vi "Async Engine.vi"(10 "Parameters":variant, 11 "Process":refnum<class "Process.lvclass">) -> ()   [LabVIEW 2019, in "Fuel Injector Analysis Addon Engine.lvlib"]
uses:
  Fuel Injector Analysis Addon Engine.lvlib
  <vilib>/NI/NIVS Inline Async API/_VS Inline Async API/Process/Process.lvclass
  Addon Shared/Types/Injector info.ctl
  Addon Shared/Fuel Injector Analysis Addon Shared.lvlib
  <vilib>/NI VeriStand/Custom Device API/Waveform Data Reference.ctl
  <vilib>/NI VeriStand/Custom Device API/Custom Device API.lvlib
  <vilib>/NI VeriStand/Custom Device Waveform API/Single Waveform Write (DBL)/Single Waveform Write (DBL).lvclass
  Types/Async Parameters.ctl
  <vilib>/NI/NIVS Inline Async API/_Data Access Engine/Data Access Engine/Data Access Engine.lvclass
  <vilib>/Platform/TimedLoop/XDataNode/XDataNode.xnode
  <vilib>/Platform/TimedLoop/XDataNode/nitl_modes.ctl
  <vilib>/Platform/TimedLoop/XDataNode/XDNodeRunTimeDep.lvlib
  <vilib>/Platform/TimedLoop/XDataNode/wakeup.ctl
  <vilib>/Platform/TimedLoop/XDataNode/timing_clust.ctl
  Addon Shared/Constants.vi
  <vilib>/NI/NIVS Inline Async API/_Data Access Engine/Access Type Classes/Read/Read.lvclass
  <vilib>/NI/NIVS Inline Async API/_Data Access Engine/Access Type Classes/Write/Write.lvclass
  <vilib>/NI/NIVS Inline Async API/_Data Access Engine/Data Access Engine/Methods/Write.Lookup.vi
  Addon Shared/Types/Analysis.Channels.Select.ctl
  <vilib>/NI/NIVS Inline Async API/_Data Access Engine/Data Access Engine/Methods/Read.Lookup.vi
  <vilib>/NI/NIVS Inline Async API/_Data Access Engine/Data Access Engine/Types/Write.DVR.ctl
  <vilib>/NI/NIVS Inline Async API/_Data Access Engine/Data Access Engine/Types/Read.DVR.ctl
  Addon Shared/Types/Stage.Transition.Types.ctl
  Addon Shared/Types/Stage.PullIn.Types.ctl
  Addon Shared/Types/Stage.Parameters.ctl
  Addon Shared/Types/Shot.Parameters.ctl
  Types/Injector.State.ctl
  Addon Shared/Types/Compiled.Group.WaveformRefs.ctl
  <vilib>/NI/NIVS Inline Async API/_Data Access Engine/Data Access Engine/Methods/Write.Data.vi
panel:
  in  "Error":errorcluster
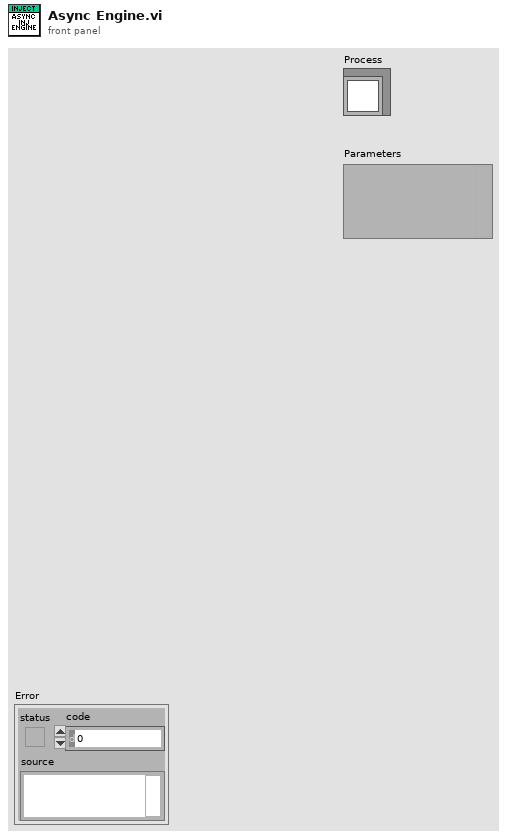
[diagram p1: front panel]
types:
  T1 = typedef "Fuel Injector Analysis Addon Engine.lvlib/Async Parameters.ctl" = cluster{"Name":string, "Injectors.Count":u8, "Groups.Settings":T2[], "Groups.InitResults":cluster{"Values":dbl[]}[], "Injectors.Settings":T7[], "Injectors.State":T8[], "DMA.Ref":refnum<k20>, "FPGA.Status":T9, "Search.Data":T10, "Results.Data":T9, "Waveform.Enable":T10, "Waveform.Refs":T11[], "Waveform.Sessions":refnum<class "Single Waveform Write (DBL).lvclass">[]}
  T2 = typedef "Fuel Injector Analysis Addon Shared.lvlib/Shot.Parameters.ctl" = cluster{"Shots":u32, "Shot.InitialVoltage":dbl, "Shot.Stages":u32, "Stages":T3[], "Timeout":dbl, "Results.Count":i32, "Active Edge":bool, "Rate.Hz":u32, "Channels":u32}
  T3 = typedef "Fuel Injector Analysis Addon Shared.lvlib/Stage.Parameters.ctl" = cluster{"Stage.Dwell.Level":dbl, "PullIn.Type":T4, "PullIn.Level":dbl, "Transition.Type":T5, "Transition.Level":dbl, "Results":T6}
  T4 = typedef "Fuel Injector Analysis Addon Shared.lvlib/Stage.PullIn.Types.ctl" = enum8{"Pull In Transition Pulses", "Pull In Transition Current Drop"}
  T5 = typedef "Fuel Injector Analysis Addon Shared.lvlib/Stage.Transition.Types.ctl" = enum8{"Stage Transition Inactive Time", "Stage Transition Voltage Increase", "Stage Transition Current Decrease", "Stage Transition Active Time"}
  T6 = typedef "Fuel Injector Analysis Addon Shared.lvlib/Analysis.Channels.Select.ctl" = cluster{"Pull In Time":bool, "Pull In Max Current":bool, "Pull In Max Voltage":bool, "Pull In Min Voltage":bool, "Pull In Avg Voltage":bool, "Hold Time":bool, "Hold Max Current":bool, "Hold Min Current":bool, "Hold Avg Current":bool, "Hold Max Voltage":bool, "Hold Min Voltage":bool, "Hold Avg Max Voltage":bool, "Hold Avg Min Voltage":bool, "Off Time":bool, "Off Max Current":bool, "Off Min Current":bool, "Off Avg Current":bool, "Off Max Voltage":bool, "Off Min Voltage":bool, "Off Avg Voltage":bool, "Total Voltage Pulses":bool, "Total Stage Time":bool}
  T7 = typedef "Fuel Injector Analysis Addon Shared.lvlib/Injector info.ctl" = cluster{"Results Index":i32, "Waveform Index":i32, "Group":u16}
  T8 = typedef "Fuel Injector Analysis Addon Engine.lvlib/Injector.State.ctl" = cluster{"Timer":u32, "Events":u64}
  T9 = typedef "Data Access Engine.lvlib/Data Access Engine.lvclass/Write.DVR.ctl" = refnum<data-value>
  T10 = typedef "Data Access Engine.lvlib/Data Access Engine.lvclass/Read.DVR.ctl" = refnum<data-value>
  T11 = typedef "Fuel Injector Analysis Addon Shared.lvlib/Compiled.Group.WaveformRefs.ctl" = cluster{"WaveformRefs":T12[], "Group":i32}
  T12 = typedef "Custom Device API.lvlib/Waveform Data Reference.ctl" = i32
  T13 = typedef "Fuel Injector Analysis Addon Engine.lvlib/Injector Event Data Cluster.ctl" = cluster{"Injector.Current":i16, "Injection.Period":dbl, "Measurements":cluster{"Shots":T14[]}[], "Shots.Count":i32, "Current.Values":dbl[], "Voltage.Values":dbl[], "Injector.Group":i16}
  T14 = typedef "Fuel Injector Analysis Addon Engine.lvlib/Shot Information Control.ctl" = cluster{"Transition.Array":i32[], "Stages.Found":u16, "Results":T15[], "Shot.Time":dbl}
  T15 = typedef "Fuel Injector Analysis Addon Engine.lvlib/Stage.Measurements.ctl" = cluster{"Pull-In Time (us)":dbl, "Pull-In Max Current":dbl, "Pull-In Max Voltage":dbl, "Pull-In Min Voltage":dbl, "Pull-In Avg Volt":dbl, "Hold-In Time (us)":dbl, "Hold-In Max Current":dbl, "Hold-In Min Current":dbl, "Hold-In Avg Current":dbl, "Hold-In Max Volt":dbl, "Hold-In Min Volt":dbl, "Hold-In Avg Max Volt":dbl, "Hold-In Avg Min Volt":dbl, "Off-Stage Time (us)":dbl, "Off-Stage Max Current":dbl, "Off-Stage Min Current":dbl, "Off-Stage Avg Current":dbl, "Off-Stage Max Volt":dbl, "Off-Stage Min Volt":dbl, "Off-Stage Avg Volt":dbl, "Total Voltage Pulses":dbl, "Total Stage Time (us)":dbl}
  T16 = typedef "XDNodeRunTimeDep.lvlib/timing_clust.ctl" = cluster{"Expected End [f-1]":u64, "Actual End [f-1]":u64, "Finished Late? [f-1]":bool, "Expected End [i-1]":u64, "Actual End [i-1]":u64, "Finished Late? [i-1]":bool, "Expected Start [i]":u64, "Actual Start [i]":u64, "Expected Start [f]":u64, "Actual Start [f]":u64, "Source Name":string, "Structure Name":string, "Period":i64, "Deadline":i64, "Offset":i64, "Start":i64, "Priority":i32, "Timeout":i32, "Mode":T17, "Wakeup Reason":T18, "Error":errorcluster, "Source Type":string, "Secondary Source Type":string, "Global End Time":u64, "Global Start Time":u64, "Frame Duration":u64, "Iteration Duration":u64, "Assigned CPU":i32, "I/O Scan Engine Mode":u32}
  T17 = typedef "XDNodeRunTimeDep.lvlib/nitl_modes.ctl" = enum32{"No Change", "Process missed periods, maintain original phase", "Discard missed periods, maintain original phase", "Process missed periods, ignore original phase", "Discard missed periods, ignore original phase"}
  T18 = typedef "XDNodeRunTimeDep.lvlib/wakeup.ctl" = enum32{"Normal", "Aborted", "Asynchronous wakeup", "Timing source error", "Timed loop error", "Timeout"}
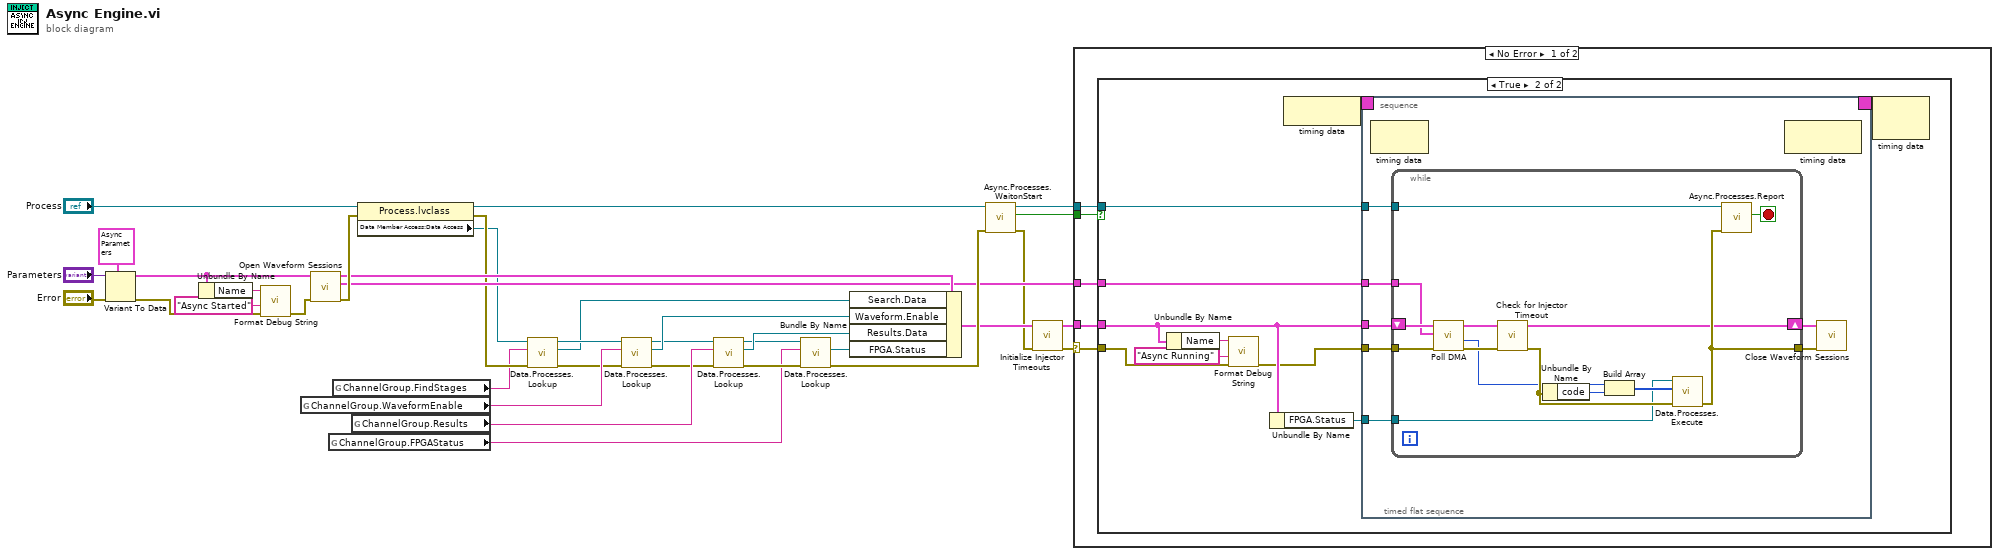
[diagram p0: block diagram]
diagram:
  n1 = Variant To Data(error in="Error", type=T1 {"Name"="", "Injectors.Count"=0, "Groups.Settings"=[], "Groups.InitResults"=[], "Injectors.Settings"=[], "Injectors.State"=[], "DMA.Ref"=refnum, "FPGA.Status"=refnum, "Search.Data"=refnum, "Results.Data"=refnum, "Waveform.Enable"=refnum, "Waveform.Refs"=[], "Waveform.Sessions"=[]} ("Parameters"), Variant="Parameters") -> (data=w4:T1, error out=w6:errorcluster)
  n2 = Unbundle By Name(w4) -> ("Name"=w3:string)
  n3 = call "Format Debug String.vi"("error in (no error)"=w6, "State"="Async Started", "Name"=w3) -> ("error out"=w5:errorcluster)  [unwired: 8 in]
  n4 = global read "Constants.vi" "ChannelGroup.WaveformEnable"() -> (w30:string)
  n5 = call "Open Waveform Sessions.vi"("error in"=w5, "Parameters"=w4) -> ("error out"=w32:errorcluster, "Injection.Results"=w18:T13, "Parameters"=w31:T1)  [unwired: 7 in]
  n6 = global read "Constants.vi" "ChannelGroup.FPGAStatus"() -> (w20:string)
  n7 = global read "Constants.vi" "ChannelGroup.FindStages"() -> (w9:string)
  n8 = global read "Constants.vi" "ChannelGroup.Results"() -> (w28:string)
  n9 = property class="Process.lvclass"(reference="Process", error in=w32) -> (reference out=w33:refnum<class "Process.lvclass">, error out=w13:errorcluster, "Data Member Access:Data Access"=w11:refnum<class "Data Access Engine.lvclass">)
  n10 = call-poly <vilib>:"Data.Processes.Lookup.vi"("error in (no error)"=w13, "Name"=w9, "Data Access API in"=w11) -> ("error out"=w12:errorcluster, "Ref"=w8:T10, "Data Access API out"=w10:refnum<class "Data Access Engine.lvclass">)  [unwired: 5 in, 1 out]
  n11 = call-poly <vilib>:"Data.Processes.Lookup.vi"("error in (no error)"=w12, "Name"=w30, "Data Access API in"=w10) -> ("error out"=w26:errorcluster, "Ref"=w29:T10, "Data Access API out"=w27:refnum<class "Data Access Engine.lvclass">)  [unwired: 5 in, 1 out]
  n12 = call-poly <vilib>:"Data.Processes.Lookup.vi"("error in (no error)"=w26, "Name"=w28, "Data Access API in"=w27) -> ("error out"=w22:errorcluster, "Ref"=w25:T9, "Data Access API out"=w23:refnum<class "Data Access Engine.lvclass">)  [unwired: 5 in, 1 out]
  n13 = call-poly <vilib>:"Data.Processes.Lookup.vi"("error in (no error)"=w22, "Name"=w20, "Data Access API in"=w23) -> ("error out"=w21:errorcluster, "Ref"=w19:T9)  [unwired: 5 in, 2 out]
  n14 = Bundle By Name(cluster=w31, "Search.Data"=w8, "Waveform.Enable"=w29, "Results.Data"=w25, "FPGA.Status"=w19) -> (w16:T1)
  n15 = call <vilib>:"Async.Processes.WaitonStart.vi"("error in (no error)"=w21, "Process"=w33) -> ("error out"=w15:errorcluster, "Execute"=w1:bool, "Process out"=w24:refnum<class "Process.lvclass">)  [unwired: 7 in]
  n16 = call "Initialize Injector Timeouts.vi"("error in (no error)"=w15, "Parameters"=w16) -> ("error out"=w14:errorcluster, "Parameters"=w17:T1)  [unwired: 8 in]
  n17 = case shown="No Error" w14 {
    selector: w14 -> [w39 _]
    tunnel: w17 -> [w38 _]
    tunnel: w24 -> [w41 _]
    tunnel: w18 -> [w40 _]
    tunnel: w1 -> [w37 _]
    frame No Error {
      n18 = case shown="True" w37 {
        tunnel: w41 -> [_ w49]
        tunnel: w40 -> [_ w45]
        tunnel: w39 -> [_ w42]
        tunnel: w38 -> [_ w44]
        frame False {
        }
        frame True {
          n19 = Unbundle By Name(w44) -> ("Name"=w47:string)
          n20 = call "Format Debug String.vi"("error in (no error)"=w42, "State"="Async Running", "Name"=w47) -> ("error out"=w43:errorcluster)  [unwired: 8 in]
          n21 = Unbundle By Name(w44) -> ("FPGA.Status"=w48:T9)
          n22 = node-c288() -> (w51:T16)
          n23 = timed-sequence {
            timing: w51 -> [_]
            timing-out: [_] -> w50
            tunnel: w44 -> [w56]
            tunnel: w43 -> [w55]
            tunnel: w49 -> [w54]
            tunnel: w45 -> [w53]
            tunnel: w48 -> [w52]
            n24 = timed-flat-sequence {
              tunnel: w56 -> [w63]
              tunnel: w55 -> [w60]
              tunnel: w54 -> [w59]
              tunnel: w53 -> [w58]
              tunnel: w52 -> [w57]
              n25 = node-c288() -> ()  [unwired: 1 in, 1 out]
              n26 = while {
                tunnel: w60 -> [w77]
                shift-right: [w70] -> w61
                shift-left: w63 -> [w68]
                tunnel: [w72] -> w62
                tunnel: w59 -> [w76]
                tunnel: w58 -> [w64]
                tunnel: w57 -> [w65]
                stop <- w75 stop-if-true
                n27 = call "Poll DMA.vi"("error in"=w77, "Injection.Results"=w64, "Parameters"=w68) -> ("error out"=w69:errorcluster, "Elements Remaining"=w67:u32, "Parameters"=w66:T1)  [unwired: 6 in]
                n28 = call "Check for Injector Timeout.vi"("error in (no error)"=w69, "Parameters"=w66) -> ("error out"=w71:errorcluster, "Parameters"=w70:T1)  [unwired: 8 in]
                n29 = Unbundle By Name(w71) -> ("code"=w73:i32)
                n30 = Build Array(w67, w73) -> (w74:u32[])
                n31 = call-poly <vilib>:"Data.Processes.Execute.vi"("error in (no error)"=w71, "Values"=w74, "Ref"=w65) -> ("error out"=w72:errorcluster)  [unwired: 8 in]
                n32 = call <vilib>:"Async.Processes.Report.vi"("Error"=w72, "Process in"=w76) -> ("Stop"=w75:bool)  [unwired: 8 in, 1 out]
              }
              n33 = node-c288() -> ()  [unwired: 1 in, 1 out]
              n34 = call "Close Waveform Sessions.vi"("error in"=w62, "Async Parameters"=w61) -> ()  [unwired: 9 in, 1 out]
            }
          }
          n35 = node-c288(w50) -> ()  [unwired: 1 out]
        }
      }
    }
    frame Error {
    }
  }
